vi "read Merkers.vi"(0 "TCP Network Connection in":refnum<k5>, 1 "U16?":bool, 5 "MW LETTURE":T2(array[cluster]), 7 "M REAL LETTURE":cluster{"MD":i16, "Descrizione":string}[](array[cluster]), 9 "M BIT LETTURE":cluster{"M":i16, "BIT":i16[]}[](array[cluster]), 11 "error in (no error)":errorcluster) -> (4 "TCP Network Connection out":refnum<k5>, 6 "MW":dbl[](array[numeric]), 8 "Array M bit":bool[](array[boolean]), 10 "M Real":dbl[](array[numeric]), 15 "error out":errorcluster)   [LabVIEW 2019]
uses:
  SIEMENS/S7Com_Source/S7Com_Data_Array.ctl
  SIEMENS/S7Com_Source/S7Com_RW_CMD.ctl
  SIEMENS/S7Com_Source/S7Com_Address_Area.ctl
  SIEMENS/S7Com_Source/S7Com_Start_Add.ctl
  SIEMENS/S7Com_Source/S7Com_Transport_Size.ctl
  SIEMENS/S7Com_Source/S7Com_Function.ctl
panel:
  out "Read_Data":T1
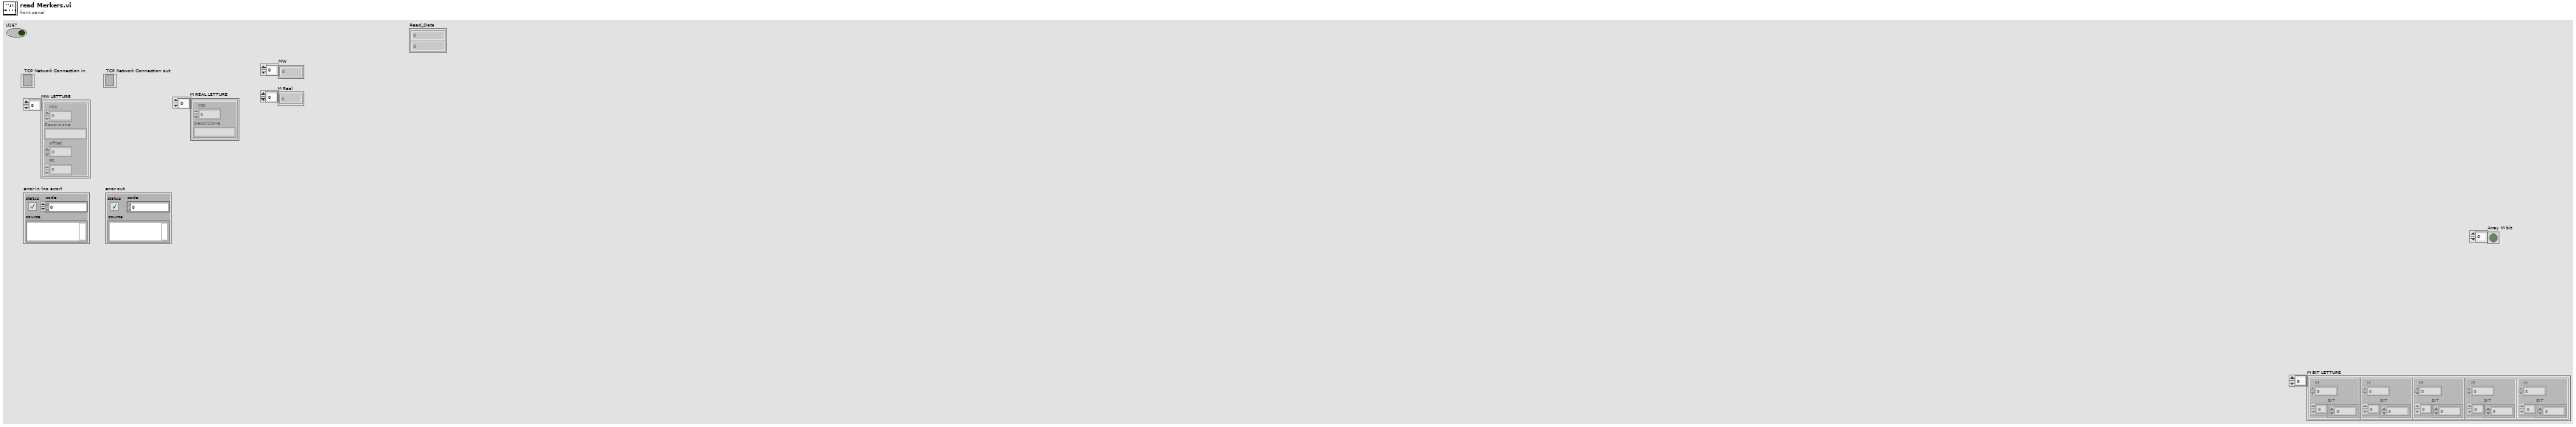
[diagram p1: front panel]
types:
  T1 = typedef "S7Com_Data_Array.ctl" = i32[]
  T2 = cluster{"MW":dbl, "Descrizione":string, "offset":dbl, "FS":dbl}[]
  T3 = typedef "S7Com_RW_CMD.ctl" = cluster{"Read Length":u16, "Data Block #":u16, "S7_Add_Area":T4, "Start Address":T5, "S7_Transport_Size":T6, "S7_Function":T7}
  T4 = typedef "S7Com_Address_Area.ctl" = u8
  T5 = typedef "S7Com_Start_Add.ctl" = u16
  T6 = typedef "S7Com_Transport_Size.ctl" = u8
  T7 = typedef "S7Com_Function.ctl" = u8
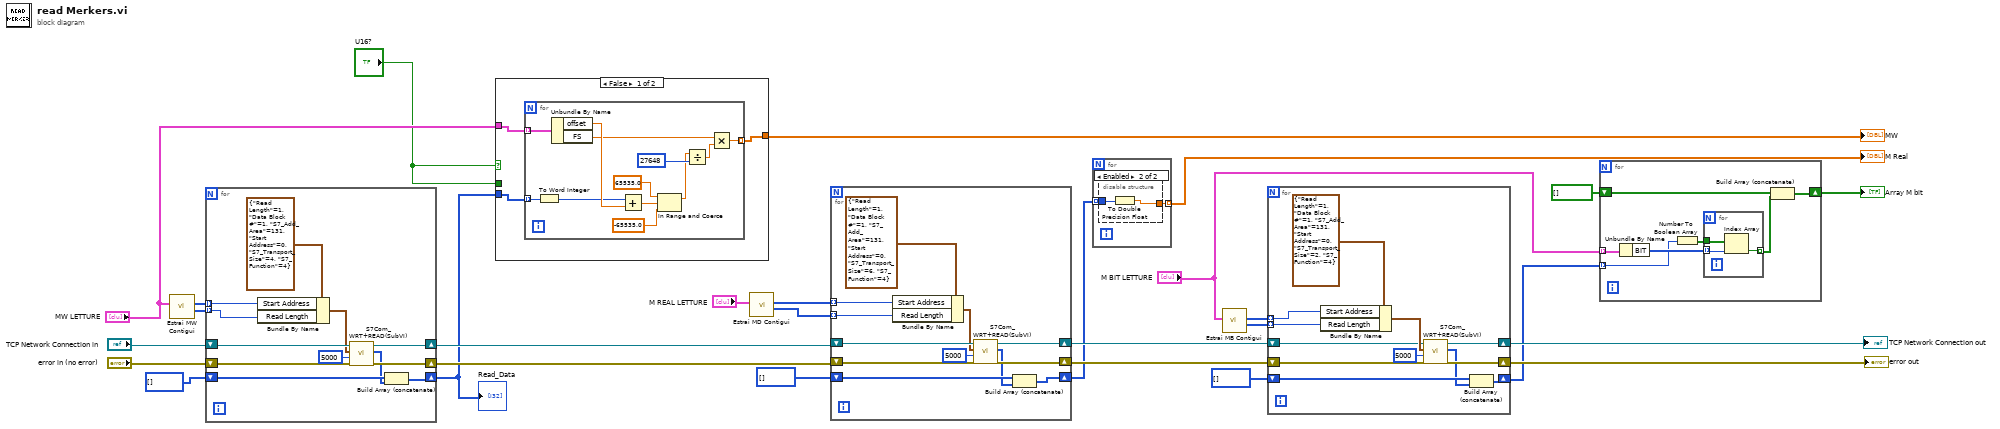
[diagram p0: block diagram]
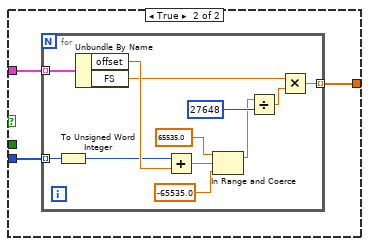
[diagram p2: hidden frame]
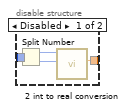
[diagram p3: hidden frame]
diagram:
  n1 = call "Estrai MW Contigui.vi"("MW LETTURE"="MW LETTURE") -> ("Number MW"=w19:i32[], "ArrayMW"=w20:i32[])  [unwired: 9 in]
  n2 = for {
    shift-right: [w36] -> w25
    shift-left: "error in (no error)" -> [w37]
    shift-right: [w38] -> w26
    shift-left: "TCP Network Connection in" -> [w39]
    tunnel: w20 -> [w33] mode=indexing
    tunnel: w19 -> [w32] mode=indexing
    shift-right: [w29] -> w15
    shift-left: T1 [] ("Read_Data") -> [w31]
    n3 = Bundle By Name(cluster=T3 {"Read Length"=1, "Data Block #"=1, "S7_Add_Area"=131, "Start Address"=0, "S7_Transport_Size"=4, "S7_Function"=4} ("RW_CMD"), "Start Address"=w33, "Read Length"=w32) -> (w35:T3)
    n4 = call "S7Com_WRT+READ(SubVI).vi"("error in"=w37, "timeout ms (25000)"=5000, "RW_CMD"=w35, "connection ID in"=w39) -> ("error out"=w36:errorcluster, "Read_Data"=w30:T1, "connection ID out"=w38:refnum<k5>)  [unwired: 1 in, 1 out]
    n5 = Build Array (concatenate)(w31, w30) -> (w29:T1)
  }
  "Read_Data" <- w15
  n6 = case shown="False" "U16?" {
    tunnel: "MW LETTURE" -> [w43 w58]
    tunnel: [w41 w57] -> w17
    tunnel: w15 -> [w42 w56]
    tunnel: "U16?" -> [_ _]
    frame False {
      n7 = for {
        tunnel: w43 -> [w55] mode=indexing
        tunnel: [w51] -> w41 mode=indexing
        tunnel: w42 -> [w45] mode=indexing
        n8 = To Word Integer(number=w45) -> (16bit integer=w44:i16)
        n9 = Unbundle By Name(w55) -> ("offset"=w54:dbl, "FS"=w52:dbl)
        n10 = Add(x=w44, y=w54) -> (x+y=w50:dbl)
        n11 = In Range and Coerce(upper limit=65535.0, x=w50, lower limit=-65535.0) -> (coerced(x)=w47:dbl)  [unwired: 1 out]
        n12 = Divide(x=w47, y=i16 27648) -> (x/y=w53:dbl)
        n13 = Multiply(x=w52, y=w53) -> (x*y=w51:dbl)
      }
    }
    frame True {
      n14 = for {
        tunnel: w58 -> [w70] mode=indexing
        tunnel: [w66] -> w57 mode=indexing
        tunnel: w56 -> [w60] mode=indexing
        n15 = To Unsigned Word Integer(number=w60) -> (unsigned 16bit integer=w59:u16)
        n16 = Unbundle By Name(w70) -> ("offset"=w69:dbl, "FS"=w67:dbl)
        n17 = Add(x=w59, y=w69) -> (x+y=w65:dbl)
        n18 = In Range and Coerce(upper limit=65535.0, x=w65, lower limit=-65535.0) -> (coerced(x)=w62:dbl)  [unwired: 1 out]
        n19 = Divide(x=w62, y=i16 27648) -> (x/y=w68:dbl)
        n20 = Multiply(x=w67, y=w68) -> (x*y=w66:dbl)
      }
    }
  }
  "MW" <- w17
  n21 = call "Estrai MD Contigui.vi"("M REAL LETTURE"="M REAL LETTURE") -> ("Number MD"=w12:i32[], "ArrayMD"=w13:i32[])  [unwired: 9 in]
  n22 = for {
    shift-right: [w78] -> w23
    shift-left: w25 -> [w79]
    shift-right: [w80] -> w24
    shift-left: w26 -> [w81]
    tunnel: w13 -> [w75] mode=indexing
    tunnel: w12 -> [w74] mode=indexing
    shift-right: [w71] -> w10
    shift-left: T1 [] ("Read_Data") -> [w73]
    n23 = Bundle By Name(cluster=T3 {"Read Length"=1, "Data Block #"=1, "S7_Add_Area"=131, "Start Address"=0, "S7_Transport_Size"=6, "S7_Function"=4} ("RW_CMD"), "Start Address"=w75, "Read Length"=w74) -> (w77:T3)
    n24 = call "S7Com_WRT+READ(SubVI).vi"("error in"=w79, "timeout ms (25000)"=5000, "RW_CMD"=w77, "connection ID in"=w81) -> ("error out"=w78:errorcluster, "Read_Data"=w72:T1, "connection ID out"=w80:refnum<k5>)  [unwired: 1 in, 1 out]
    n25 = Build Array (concatenate)(w73, w72) -> (w71:T1)
  }
  n26 = for {
    tunnel: [w84] -> w9 mode=indexing
    tunnel: w10 -> [w83] mode=indexing
    n27 = disable-structure shown="Enabled" {
      disable-tunnel: [w86 w89] -> w84
      disable-tunnel: w83 -> [w85 w90]
      frame Disabled {
        n28 = Split Number(x=w85) -> (hi(x)=w88:u16, lo(x)=w87:u16)
        n29 = call "2 int to real conversion.vi"("MW 15 0 in"=w87, "MW 31 16 in"=w88) -> ("reale out"=w86:dbl)  [unwired: 7 in, 2 out]
      }
      frame Enabled {
        n30 = To Double Precision Float(number=w90) -> (double precision float=w89:dbl)
      }
    }
  }
  "M Real" <- w9
  n31 = call "Estrai MB Contigui.vi"("M BIT LETTURE"="M BIT LETTURE") -> ("Number MB"=w6:i32[], "ArrayMB"=w7:i32[])  [unwired: 9 in]
  n32 = for {
    shift-right: [w97] -> w22
    shift-left: w23 -> [w98]
    shift-right: [w99] -> w21
    shift-left: w24 -> [w100]
    tunnel: w7 -> [w95] mode=indexing
    tunnel: w6 -> [w94] mode=indexing
    shift-right: [w91] -> w4
    shift-left: T1 [] ("Read_Data") -> [w93]
    n33 = Bundle By Name(cluster=T3 {"Read Length"=1, "Data Block #"=1, "S7_Add_Area"=131, "Start Address"=0, "S7_Transport_Size"=2, "S7_Function"=4} ("RW_CMD"), "Start Address"=w95, "Read Length"=w94) -> (w102:T3)
    n34 = call "S7Com_WRT+READ(SubVI).vi"("error in"=w98, "timeout ms (25000)"=5000, "RW_CMD"=w102, "connection ID in"=w100) -> ("error out"=w97:errorcluster, "Read_Data"=w92:T1, "connection ID out"=w99:refnum<k5>)  [unwired: 1 in, 1 out]
    n35 = Build Array (concatenate)(w93, w92) -> (w91:T1)
  }
  "TCP Network Connection out" <- w21
  "error out" <- w22
  n36 = for {
    tunnel: "M BIT LETTURE" -> [w109] mode=indexing
    shift-right: [w104] -> w3
    shift-left: bool[] [] -> [w105]
    tunnel: w4 -> [w103] mode=indexing
    n37 = Unbundle By Name(w109) -> ("BIT"=w108:i16[])
    n38 = Number To Boolean Array(number=w103) -> (Boolean array=w107:bool[])
    n39 = for {
      tunnel: w108 -> [w112] mode=indexing
      tunnel: w107 -> [w111]
      tunnel: [w110] -> w106 mode=indexing
      n40 = Index Array(array=w111, index=w112) -> (element=w110:bool)
    }
    n41 = Build Array (concatenate)(w105, w106) -> (w104:bool[])
  }
  "Array M bit" <- w3
